vi "create Renderer.vi"(5 "pMaxTextureHeight":i32, 6 "pMaxTextureWidth":i32, 7 "pBytesPerVoxel":i32, 8 "error in (no error)":errorcluster, 9 "pWindowHeight":i32, 10 "pWindowWidth":i32, 11 "pRendererId":i32) -> (0 "error out":errorcluster, 3 "function return":i32)   [LabVIEW 2012, in "clearvolume.lvlib"]
doc: "__declspec(dllexport) long __cdecl createRenderer( int pRendererId,\n int pWindowWidth,\n int pWindowHeight,\n int pBytesPerVoxel,\n int pMaxTextureWidth,\n int pMaxTextureHeight);"
uses:
  clearvolume.lvlib
  clearvolume.dll
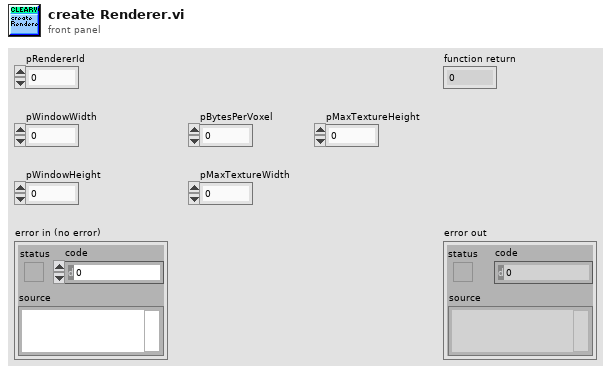
[diagram p1: front panel]
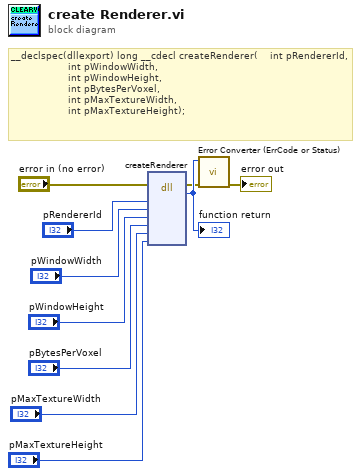
[diagram p0: block diagram]
diagram:
  # "__declspec(dllexport) long __cdecl createRenderer(\t\t\t\tint pRendererId,\n\t\t\t\t\t\t\t\t\t\t\t\t\t\t\t\t\t\t\tint pWindowWidth,\n\t\t\t\t\t\t\t\t\t\t\t\t\t\t\t\t\t\t\tint pWindowHeight,\n\t\t\t\t\t\t\t\t\t\t\t\t\t\t\t\t\t\t\tint pBytesPerVoxel,\n\t\t\t\t\t\t\t\t\t\t\t\t\t\t\t\t\t\t\tint pMaxTextureWidth,\n\t\t\t\t\t\t\t\t\t\t\t\t\t\t\t\t\t\t\tint pMaxTextureHeight);"
  n1 = dll-call lib="C:/Users/myerslab/workspace/Libraries/CV/clearvolume/src/labview/clearvolume/clearvolume.*" fn="createRenderer"(error in="error in (no error)", "pRendererId"="pRendererId", "pWindowWidth"="pWindowWidth", "pWindowHeight"="pWindowHeight", "pBytesPerVoxel"="pBytesPerVoxel", "pMaxTextureWidth"="pMaxTextureWidth", "pMaxTextureHeight"="pMaxTextureHeight") -> (error out=w2:errorcluster, w10:i32)  [unwired: 8 in, 1 out]
  "function return" <- w10
  n2 = call "Error Converter (ErrCode or Status).vi"("error in (no error)"=w2, "error code"=w10) -> ("error out"=→"error out":errorcluster)  [unwired: 9 in]
